vi "RFID更新 - 副本.vi"(2 "随形板ID":string, 4 "壳体码":string) -> ()   [LabVIEW 2013]
uses:
  <vilib>/Utility/error.llb/whitespace.ctl
panel:
  in  "error in (no error)":errorcluster
  out "error out":errorcluster
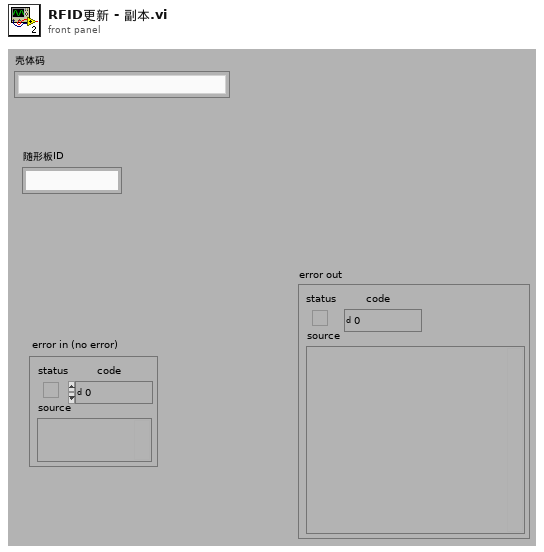
[diagram p1: front panel]
types:
  T1 = typedef "whitespace.ctl" = u16
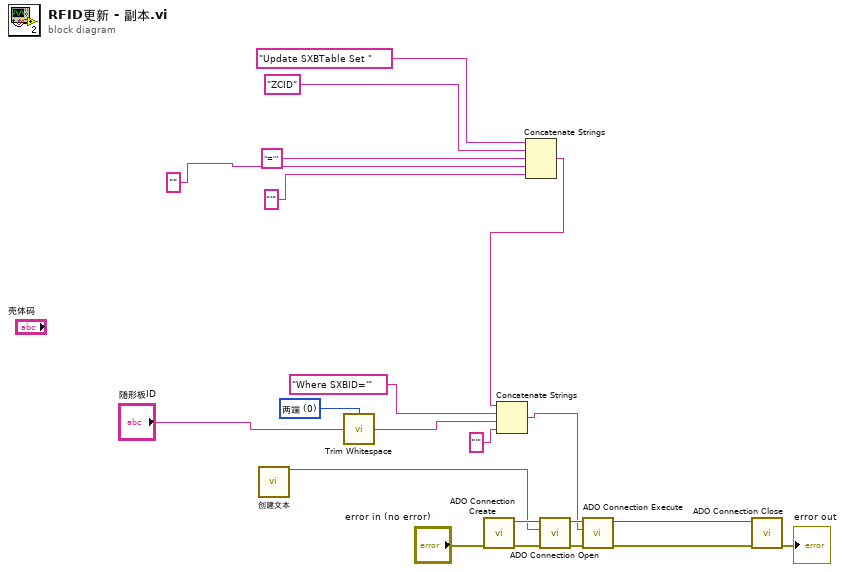
[diagram p0: block diagram]
diagram:
  w13 = T1 0 items=["两端", "字符串首端", "字符串末端"] ("location (both)")
  n1 = call "创建文本"() -> ("Result"=w9:string)  [unwired: 14 in, 1 out]
  n2 = call <vilib>:"Trim Whitespace.vi"("string"="随形板ID", "location (both)"=w13) -> ("trimmed string"=w11:string)
  n3 = call "ADO Connection Create.vi"("error in (no error)"="error in (no error)") -> ("error out"=w20:errorcluster, "ADODB._Connection Out"=w21:refnum<k7>)  [unwired: 9 out]
  n4 = Concatenate Strings("Update SXBTable Set " ("字符串"), "ZCID", "='", "" ("字符串"), "'" ("字符串")) -> (w3:string)
  n5 = Concatenate Strings(w3, "Where SXBID='" ("字符串"), w11, "'" ("字符串")) -> (w8:string)
  n6 = call "ADO Connection Open.vi"("error in (no error)"=w20, "ConnectionString"=w9, "ADODB._Connection In"=w21) -> ("error out"=w19:errorcluster, "ADODB._Connection Out"=w18:refnum<k7>)  [unwired: 7 out]
  n7 = call "ADO Connection Execute.vi"("error in (no error)"=w19, "CommandText"=w8, "ADODB._Connection In"=w18) -> ("error out"=w14:errorcluster, "ADODB._Connection Out"=w17:refnum<k7>)  [unwired: 7 out]
  n8 = call "ADO Connection Close.vi"("error in (no error)"=w14, "ADODB._Connection In"=w17) -> ("error out"=→"error out":errorcluster)  [unwired: 9 out]
